vi "Tmotor TEST.vi"() -> ()   [LabVIEW 2019]
uses:
  <vilib>/rvi/Emulation/niFpgaGetClockAttributes.vi
  <vilib>/rvi/Emulation/niFpgaSctlEmulationGetInTimedLoop.vi
  <vilib>/rvi/Emulation/niFpgaEmulationReportErrorSimple.vi
  <vilib>/rvi/Emulation/niFpgaCriticalErrorInLSC.vi
panel:
  in  "Start Up ID":u32 format="%x"
  out "Read Data?":bool
  in  "Loop Time":u32 caption="Loop Time (ms)"
  in  "stop":bool
  in  "Control Value":fxp<+/-,32,16>
  in  "Mode":enum16{"Position", "Velocity", "Torque"}(ring)
  in  "ID In":u32 format="%x"
  out "ID Out":u32
  out "Torque":fxp<+/-,32,16>
  out "Velocity":fxp<+/-,32,16>
  out "Position":fxp<+/-,32,16>
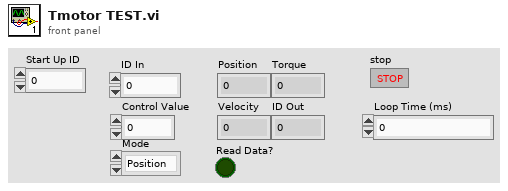
[diagram p1: front panel]
types:
  T1 = typedef "SPI Config.ctl" = cluster{"MXP Port":enum16{"A", "B"}, "Device":enum16{"CAN", "ENC", "IMU1", "IMU2"}, "CPOL":bool}
  T2 = cluster{"Position":fxp<+/-,32,16>, "Velocity":fxp<+/-,32,16>, "Torque":fxp<+/-,32,16>, "ID":u32, "Read Data?":bool}
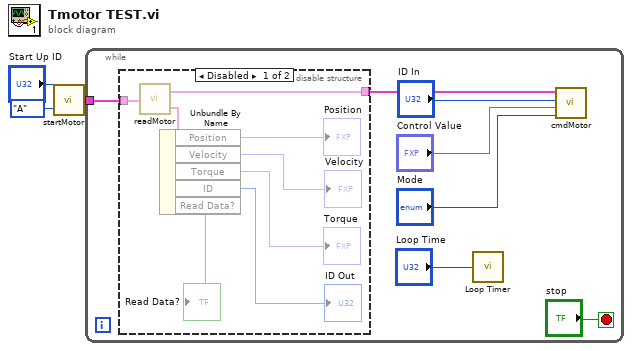
[diagram p0: block diagram]
diagram:
  n1 = call "startMotor.vi"("MXP Port"=enum16{"A", "B"}."A", "ID"="Start Up ID") -> ("SPI Config Out"=w3:T1)
  n2 = while {
    tunnel: w3 -> [w10]
    stop <- "stop" stop-if-true
    n3 = disable-structure shown="Disabled" {
      disable-tunnel: w10 -> [w18 _]
      disable-tunnel: [w17 _] -> w9
      frame Disabled {
        n4 = call "readMotor.vi"("SPI Config In"=w18) -> ("SPI Config Out"=w17:T1, "Data Out"=w16:T2)
        n5 = Unbundle By Name(w16) -> ("Position"=→"Position":fxp<+/-,32,16>, "Velocity"=→"Velocity":fxp<+/-,32,16>, "Torque"=→"Torque":fxp<+/-,32,16>, "ID"=→"ID Out":u32, "Read Data?"=→"Read Data?":bool)
      }
      frame Enabled {
      }
    }
    n6 = call "Loop Timer"("Count(mSec)"="Loop Time") -> ()  [unwired: 1 out]
    n7 = call "cmdMotor.vi"("Mode"="Mode", "Control Value"="Control Value", "ID"="ID In", "SPI Config In"=w9) -> ()  [unwired: 1 out]
  }
